vi "Connection Listener.vi"(0 "Websocket In":refnum<class "Websocket.lvclass">, 5 "error in":errorcluster) -> (14 "Websocket Out":refnum<class "Websocket.lvclass">, 19 "error out":errorcluster)   [LabVIEW 2017, in "Front Panel Publisher.lvlib" / "Websocket.lvclass"]
uses:
  Websocket.lvclass
panel:
  out "Stop":bool
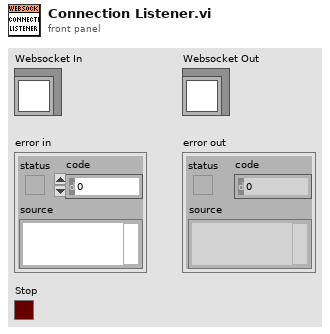
[diagram p1: front panel]
types:
  T1 = typedef "FrontPanelPublisher.lvlib/Websocket.lvclass/ObjectAttributes.ctl" = cluster{"Port":u16, "TCP Refs":refnum<k5>[], "Connection IDs":u64[]}
  T2 = enum16{"Standard", "Buffered", "CRLF", "Immediate"}
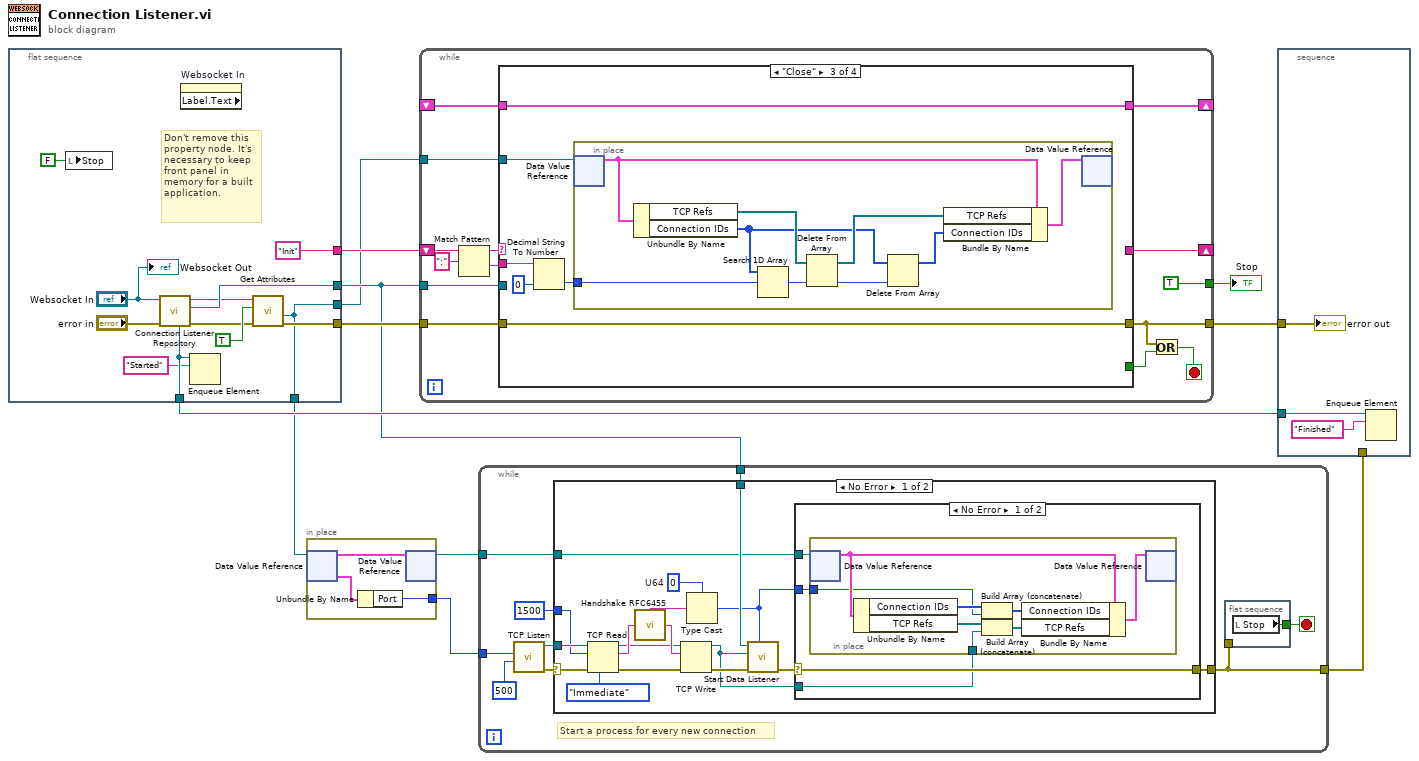
[diagram p0: block diagram]
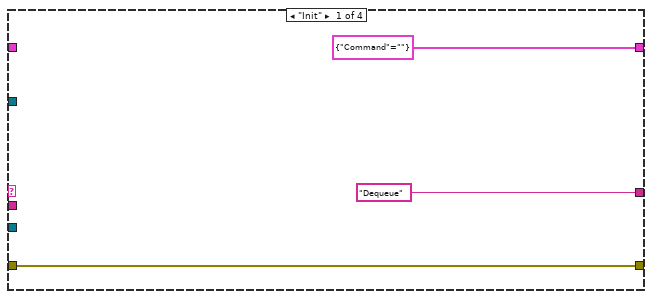
[diagram p4: hidden frame]
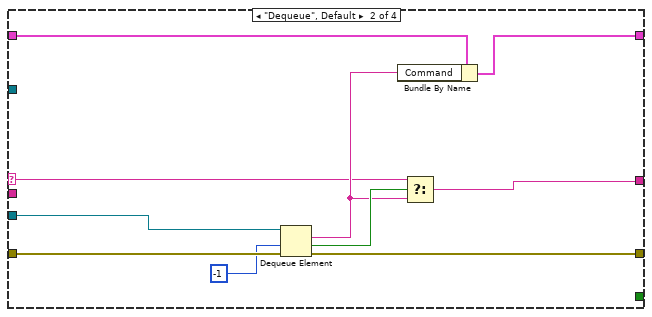
[diagram p5: hidden frame]
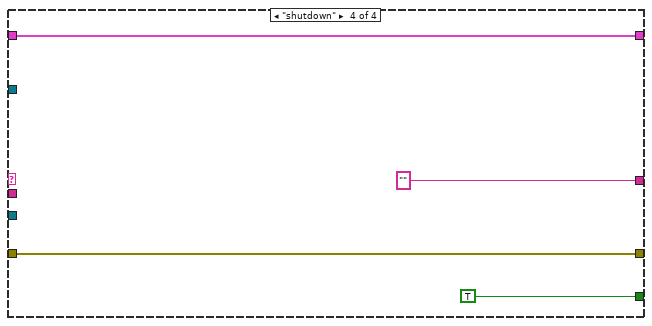
[diagram p6: hidden frame]
diagram:
  n1 = flat-sequence {
    tunnel: [w14] -> w11
    tunnel: [w23] -> w4
    tunnel: [w22] -> w9
    tunnel: ["Init"] -> w8
    tunnel: [w13] -> w6
    tunnel: [w13] -> w3
    frame #0 {
      # "Don't remove this property node. It's necessary to keep front panel in memory for a built application."
      n2 = local write "Stop"(FALSE ("Stop")) -> ()
      n3 = call "Connection Listener Repository.vi"("error in (no error)"="error in", "Websocket In"="Websocket In") -> ("error out"=w15:errorcluster, "ToProcessQueue"=w23:refnum<queue>, "Websocket Out"=w16:refnum<class "Websocket.lvclass">, "ProcessSyncQueue"=w22:refnum<queue>)  [unwired: 3 in, 3 out]
      n4 = property on="Websocket In" class="LVClassControl (strict)" props=["Label", "Text"]() -> ()  [unwired: 2 in, 3 out]
      n5 = Enqueue Element(queue=w22, element="Started") -> ()  [unwired: 2 in, 3 out]
      n6 = call "Get Attributes.vi"("error in (no error)"=w15, "Only Get DVR Reference"=TRUE ("OnlyGetDvrReference(False)"), "reference in"=w16) -> ("error out"=w14:errorcluster, "DataRef"=w13:refnum<data-value>)  [unwired: 5 in, 2 out]
      "Websocket Out" <- "Websocket In"
    }
  }
  n7 = in-place {
    in-place-border: [w24] -> w7
    n8 = in-place-dvr #1(w6) -> (w25:T1)  [unwired: 1 out]
    n9 = Unbundle By Name(w25) -> ("Port"=w24:u16)
    n10 = in-place-dvr #1(w25) -> (w2:refnum<data-value>)  [unwired: 1 out]
  }
  n11 = while {
    tunnel: w4 -> [w39]
    shift-right: [w31] -> _
    shift-left: w8 -> [w37]
    shift-right: [w34] -> _
    shift-left: _ -> [w33]
    tunnel: w11 -> [w32]
    tunnel: [w29] -> w10
    tunnel: w3 -> [w30]
    tunnel: [TRUE ("Stop")] -> w1
    stop <- w28 stop-if-true
    n12 = Match Pattern(string=w37, regular expression=":") -> (before substring=w36:string, after substring=w35:string)  [unwired: 1 in, 2 out]
    n13 = case shown="\"Close\"" w36 {
      selector: w36 -> [_ w43 _ _]
      tunnel: w32 -> [w41 w52 w56 w70]
      tunnel: [w41 w51 w56 w70] -> w29
      tunnel: w39 -> [_ w49 _ _]
      tunnel: w35 -> [_ _ w58 _]
      tunnel: ["Dequeue" ("t") w47 _ "" ("y")] -> w31
      tunnel: [cluster{"Command":string} {"Command"=""} ("LocalVariable") w44 w55 w68] -> w34
      tunnel: w33 -> [_ w45 w55 w68]
      tunnel: [_ _ _ TRUE] -> w27
      tunnel: w30 -> [_ _ w54 _]
      frame "Init" {
      }
      frame "Dequeue", Default {
        n14 = Dequeue Element(queue=w49, timeout in ms (-1)=-1, error in (no error)=w52) -> (element=w46:string, timed out?=w48:bool, error out=w51:errorcluster)  [unwired: 1 out]
        n15 = Bundle By Name(cluster=w45, "Command"=w46) -> (w44:cluster{"Command":string})
        n16 = Select(t=w43, s=w48, f=w46) -> (s? t:f=w47:string)
      }
      frame "Close" {
        n17 = Decimal String To Number(string=w58, default (0L)=u64 0 ("default (0 I32)")) -> (number=w53:u64)  [unwired: 1 in, 1 out]
        n18 = in-place {
          in-place-border: w53 -> [w64]
          n19 = in-place-dvr #2(w54) -> (w66:T1)  [unwired: 1 out]
          n20 = Unbundle By Name(w66) -> ("TCP Refs"=w63:refnum<k5>[], "Connection IDs"=w61:u64[])
          n21 = Search 1D Array(1D array=w61, element=w64) -> (index of element=w59:i32)  [unwired: 1 in]
          n22 = Delete From Array(array=w63, index=w59) -> (array with subset deleted=w62:refnum<k5>[])  [unwired: 1 in, 1 out]
          n23 = Delete From Array(array=w61, index=w59) -> (array with subset deleted=w60:u64[])  [unwired: 1 in, 1 out]
          n24 = Bundle By Name(cluster=w66, "TCP Refs"=w62, "Connection IDs"=w60) -> (w65:T1)
          n25 = in-place-dvr #2(w65) -> ()  [unwired: 2 out]
        }
      }
      frame "shutdown" {
      }
    }
    n26 = Or(x=w29, y=w27) -> (x .or. y?=w28:bool)
  }
  "Stop" <- w1
  n27 = while {
    tunnel: w7 -> [w76]
    tunnel: [w72] -> w5
    tunnel: w4 -> [w74]
    tunnel: w2 -> [w71]
    stop <- w73 stop-if-true
    # "Start a process for every new connection"
    n28 = call <vilib>:"TCP Listen.vi"("timeout ms (wait forever: -1)"=500, "port"=w76) -> ("error out"=w78:errorcluster, "connection ID"=w79:refnum<k5>)  [unwired: 5 in, 3 out]
    n29 = case shown="No Error" w78 {
      selector: w78 -> [w97 w111]
      tunnel: w79 -> [w90 _]
      tunnel: [w83 w111] -> w72
      tunnel: 1500 ("timeout ms (wait forever: -1)") -> [w88 _]
      tunnel: w74 -> [w86 _]
      tunnel: w71 -> [w85 _]
      frame No Error {
        w94 = u64 0  # U64
        n30 = TCP Read(connection ID=w90, bytes to read=w88, error in (no error)=w97, 7:T2."Immediate" ("mode (standard)")) -> (connection ID out=w89:refnum<k5>, data out=w92:string, error out=w96:errorcluster)  [unwired: 1 in]
        n31 = call "Handshake RFC6455.vi"("websocket client handshake"=w92) -> ("accept string"=w93:string, "websocket server handshake"=w95:string)
        n32 = TCP Write(connection ID=w89, data in=w95, error in (no error)=w96) -> (connection ID out=w81:refnum<k5>, error out=w87:errorcluster)  [unwired: 1 in, 1 out]
        n33 = Type Cast(type=w94, x=w93) -> (*(type *) &x=w82:u64)
        n34 = call "Start Data Listener.vi"("Connection ID"=w82, "error in (no error)"=w87, "TCP  Ref"=w81, "ConListenerQ"=w86) -> ("error out"=w84:errorcluster)  [unwired: 6 in, 1 out]
        n35 = case shown="No Error" w84 {
          selector: w84 -> [w100 w110]
          tunnel: w85 -> [w101 _]
          tunnel: [w100 w110] -> w83
          tunnel: w82 -> [w99 _]
          tunnel: w81 -> [w98 _]
          frame No Error {
            n36 = in-place {
              in-place-border: w99 -> [w103]
              in-place-border: w98 -> [w102]
              n37 = in-place-dvr #3(w101) -> (w109:T1)  [unwired: 1 out]
              n38 = Unbundle By Name(w109) -> ("Connection IDs"=w107:u64[], "TCP Refs"=w106:refnum<k5>[])
              n39 = Build Array (concatenate)(w107, w103) -> (w105:u64[])
              n40 = Build Array (concatenate)(w106, w102) -> (w104:refnum<k5>[])
              n41 = Bundle By Name(cluster=w109, "Connection IDs"=w105, "TCP Refs"=w104) -> (w108:T1)
              n42 = in-place-dvr #3(w108) -> ()  [unwired: 2 out]
            }
          }
          frame Error {
          }
        }
      }
      frame Error {
      }
    }
    n43 = flat-sequence {
      tunnel: [w80] -> w73
      tunnel: w72 -> [_]
      frame #0 {
        n44 = local read "Stop"() -> (w80:bool)
      }
    }
  }
  n45 = stacked-sequence {
    tunnel: w10 -> [w114]
    tunnel: w9 -> [w113]
    tunnel: w5 -> [_]
    frame #0 {
      n46 = Enqueue Element(queue=w113, element="Finished") -> ()  [unwired: 2 in, 3 out]
      "error out" <- w114
    }
  }
